vi "StopClone.vi"(8 "error in (no error)":errorcluster, 9 "Wait for Module to stop?":bool, 11 "ModuleAdmin":refnum<class "ModuleAdmin.lvclass">) -> (0 "error out":errorcluster)   [LabVIEW 2018, in "ScopeModule.lvlib"]
uses:
  ScopeModule.lvlib
  <userlib>/NIST/ModuleAdminLib/ModuleAdmin/ModuleAdmin.lvclass
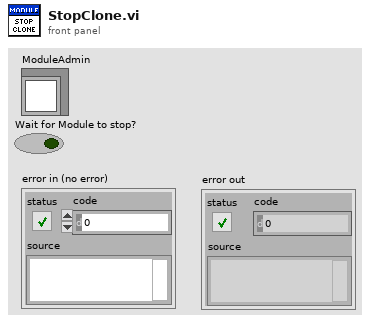
[diagram p1: front panel]
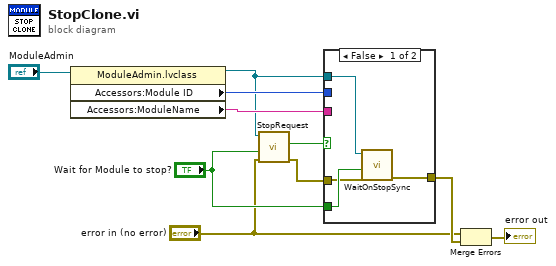
[diagram p0: block diagram]
diagram:
  n1 = property class="ModuleAdmin.lvclass"(reference="ModuleAdmin") -> (reference out=w1:refnum<class "ModuleAdmin.lvclass">, "Accessors:Module ID"=w4:i32, "Accessors:ModuleName"=w3:string)  [unwired: 1 in, 1 out]
  n2 = call "StopRequest.vi"("error in (no error)"="error in (no error)", "Wait for Module to stop? (F)"="Wait for Module to stop?", "ModuleAdmin"=w1) -> ("error out"=w5:errorcluster, "Stop Request Sent"=w6:bool)  [unwired: 7 in]
  n3 = case shown="False" w6 {
    tunnel: w4 -> [_ _]
    tunnel: w3 -> [_ _]
    tunnel: "Wait for Module to stop?" -> [w14 _]
    tunnel: [w13 w15] -> w9
    tunnel: w5 -> [w12 w15]
    tunnel: w1 -> [w11 _]
    frame False {
      n4 = call <userlib>:"WaitOnStopSync.vi"("error in (no error)"=w12, "WaitForModuleToStop?"=w14, "ModuleAdmin"=w11) -> ("error out"=w13:errorcluster)  [unwired: 7 in, 1 out]
    }
    frame True {
    }
  }
  n5 = Merge Errors("error in (no error)", w9) -> (→"error out":errorcluster)
